vi "FilterOutProbes.vi"(0 "VI reference":refnum<vi>, 1 "Exists at index":i32, 2 "Item Name":string) -> (8 "Include?":bool)   [LabVIEW 2013]
doc: "Custom probes are included in the App.AllVIs list. These entries, since they do not have a filename extension, will cause errors in the \"Compare Two Paths\" VI when it is called downstream. This VI removes the names of custom probes from the list, hence suppressing the errors.\n\n#Optimize -- There exists a VI property called \"IsProbe\". Could reading this property improve performance over parsing every VIs name?"
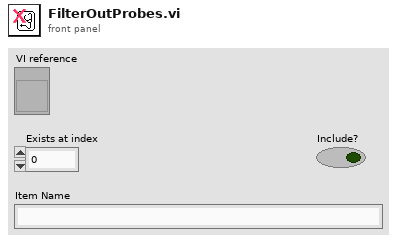
[diagram p1: front panel]
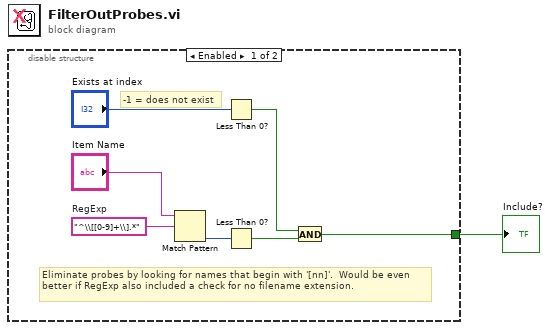
[diagram p0: block diagram]
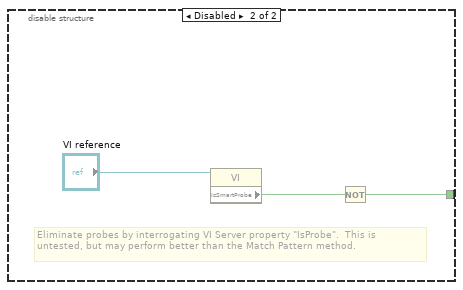
[diagram p2: hidden frame]
diagram:
  n1 = disable-structure shown="Enabled" {
    disable-tunnel: [w2 w9] -> w1
    frame Enabled {
      w5 = "^\\[[0-9]+\\].*"  # RegExp
      # "-1 = does not exist"
      # "Eliminate probes by looking for names that begin with '[nn]'.  Would be even better if RegExp also included a check for no filename extension."
      n2 = Match Pattern(string="Item Name", regular expression=w5) -> (offset past match=w6:i32)  [unwired: 1 in, 3 out]
      n3 = Less Than 0?(x="Exists at index") -> (x < 0?=w3:bool)
      n4 = Less Than 0?(x=w6) -> (x < 0?=w7:bool)
      n5 = And(x=w3, y=w7) -> (x .and. y?=w2:bool)
    }
    frame Disabled {
      # "Eliminate probes by interrogating VI Server property \"IsProbe\".  This is untested, but may perform better than the Match Pattern method."
      n6 = property class="VI"(reference="VI reference") -> ("IsSmartProbe"=w10:bool)  [unwired: 1 in, 2 out]
      n7 = Not(x=w10) -> (.not. x?=w9:bool)
    }
  }
  "Include?" <- w1
